vi "ListViews.vi"(8 "error in (no error)":errorcluster, 11 "ViewMgr in":refnum<class "ViewMgr.lvclass">) -> (0 "error out":errorcluster, 2 "names":string[](array[string]), 3 "ViewMgr out":refnum<class "ViewMgr.lvclass">)   [LabVIEW 2020, in "CSM-TagDBDisplayContainer.lvlib" / "ViewMgr.lvclass"]
uses:
  ViewMgr.lvclass
  ViewMgr.lvclass/ViewMgr.ctl
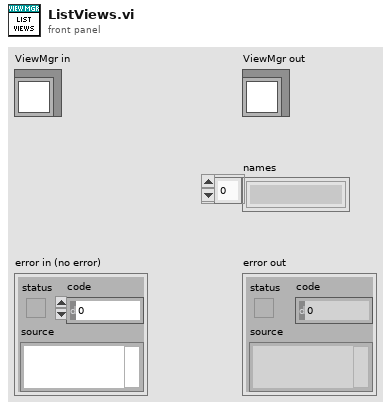
[diagram p1: front panel]
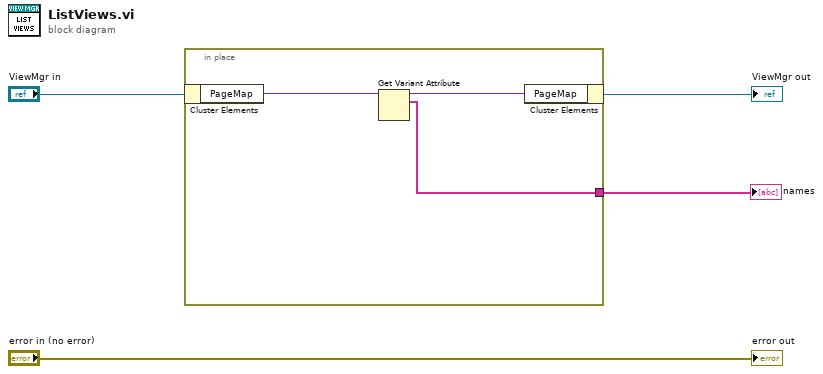
[diagram p0: block diagram]
diagram:
  n1 = in-place {
    in-place-border: [w5] -> w1
    n2 = in-place-cluster #1("ViewMgr in") -> ("PageMap"=w7:variant)
    n3 = Get Variant Attribute(Variant=w7) -> (duplicate Variant=w6:variant, names=w5:string[])  [unwired: 3 in, 2 out]
    n4 = in-place-cluster #1("PageMap"=w6) -> (→"ViewMgr out":refnum<class "ViewMgr.lvclass">)
  }
  "names" <- w1
  "error out" <- "error in (no error)"
